vi "color config.vi"(11 "color 1":T1) -> (2 "max":dbl, 3 "Array":cluster{dbl, u32}[](array[cluster]))   [LabVIEW 2018]
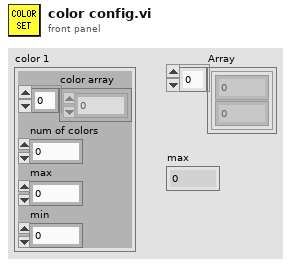
[diagram p1: front panel]
types:
  T1 = cluster{"color array":u32[], "num of colors":i32, "max":dbl, "min":dbl}
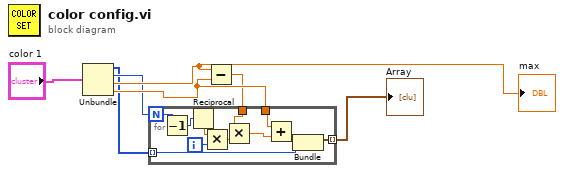
[diagram p0: block diagram]
diagram:
  n1 = Unbundle("color 1") -> ("color array"=w4:u32[], "num of colors"=w5:i32, "max"=w6:dbl, "min"=w7:dbl)
  "max" <- w6
  n2 = Subtract(x=w6, y=w7) -> (x-y=w1:dbl)
  n3 = for {
    N: w5 -> [w12]
    tunnel: w1 -> [w16]
    tunnel: [w14] -> w2 mode=indexing
    tunnel: w4 -> [w13] mode=indexing
    tunnel: w7 -> [w8]
    i -> [w18]
    n4 = Decrement(x=w12) -> (x-1=w11:i32)
    n5 = Reciprocal(x=w11) -> (1/x=w10:dbl)
    n6 = Multiply(x=w10, y=w18) -> (x*y=w17:dbl)
    n7 = Multiply(x=w16, y=w17) -> (x*y=w15:dbl)
    n8 = Add(x=w8, y=w15) -> (x+y=w9:dbl)
    n9 = Bundle(w9, w13) -> (w14:cluster{dbl, u32})  [unwired: 1 in]
  }
  "Array" <- w2
